vi "Initialize.vi"(8 "error in (no error)":errorcluster, 9 "Data Cluster (for Table Headers)":variant, 10 "TableLogger Config":T1, 11 "object in":refnum<class "TableLogger_SQLite_Actor.lvclass">) -> (0 "error out":errorcluster, 3 "object out":refnum<class "TableLogger_SQLite_Actor.lvclass">)   [LabVIEW 2014, in "TableLogger_SQLite_Actor.lvlib" / "TableLogger_SQLite_Actor.lvclass"]
uses:
  TableLogger_SQLite_Actor.lvclass
  TableLogger_Actor/TableLoggerConfig.ctl
  TableLogger_Actor/TableLoggerTypes.ctl
  TableLogger_Actor/TableLoggerBackupConfig.ctl
  TableLogger_SQLite_Actor.lvclass/TableLogger_SQLite_Actor.ctl
  <vilib>/drjdpowell/SQLite Library/SQL Connection/Open (path).vi
  <vilib>/drjdpowell/SQLite Library/SQL Connection/Open (string).vi
  <userlib>/_OpenG.lib/file/file.llb/Strip Path - Traditional__ogtk.vi
  <vilib>/AdvancedString/Path To Command Line String.vi
  <vilib>/drjdpowell/SQLite Library/SQL Connection/Execute SQL (No results).vi
  TableLogger_Actor/TableLogger_Actor/TableLogger_Actor.lvclass
  <vilib>/drjdpowell/SQLite Library/SQL Connection/Connection.lvclass
  <vilib>/drjdpowell/SQLite Library/SQLite.lvlib
  TableLogger_Actor/TableLogger_Actor.lvlib
panel:
  # "Connector Pane"
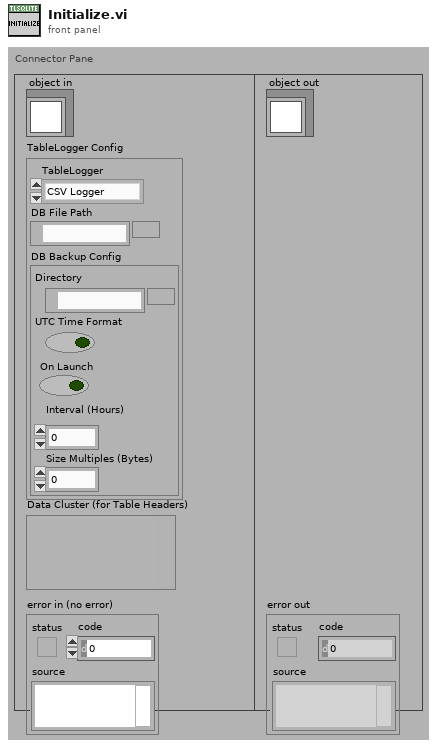
[diagram p1: front panel]
types:
  T1 = typedef "TableLogger_Actor.lvlib/TableLoggerConfig.ctl" = cluster{"TableLogger":T2, "DB File Path":path, "DB Backup Config":T3}
  T2 = typedef "TableLogger_Actor.lvlib/TableLoggerTypes.ctl" = enum16{"CSV Logger", "SQLite Logger"}
  T3 = typedef "TableLogger_Actor.lvlib/TableLoggerBackupConfig.ctl" = cluster{"Directory":path, "UTC Time Format":bool, "On Launch":bool, "Interval (Hours)":dbl, "Size Multiples (Bytes)":i32}
  T4 = typedef "Type Descriptor Enumeration__ogtk.ctl" = enum8{"<Null>", "I8", "I16", "I32", "I64", "U8", "U16", "U32", "U64", "SGL", "DBL", "EXT", "CSG", "CDB", "CXT", "0x0F", "0x10", "0x11", "0x12", "0x13", "0x14", "Enum U8", "Enum U16", "Enum U32", "Enum U64", "SGL PQ", "DBL PQ", "EXT PQ", "CSG PQ", "CDB PQ", "CXT PQ", "0x1F", "0x20", "Boolean", "0x22", "0x23", "0x24", "0x25", "0x26", "0x27", "0x28", "0x29", "0x2A", "0x2B", "0x2C", "0x2D", "0x2E", "0x2F", "String", "0x31", "Path", "Pict", "0x34", "0x35", "0x36", "DAQ", "0x38", "0x39", "0x3A", "0x3B", "0x3C", "0x3D", "0x3E", "0x3F", "Array", "0x41", "0x42", "0x43", "0x44", "0x45", "0x46", "0x47", "0x48", "0x49", "0x4A", "0x4B", "0x4C", "0x4D", "0x4E", "0x4F", "Cluster", "0x51", "0x52", "Variant", "Waveform", "0x55", "0x56", "0x57", "0x58", "0x59", "0x5A", "0x5B", "0x5C", "0x5D", "0x5E", "0x5F", "0x60", "0x61", "0x62", "0x63", "0x64", "0x65", "0x66", "0x67", "0x68", "0x69", "0x6A", "0x6B", "0x6C", "0x6D", "0x6E", "0x6F", "Refnum"}
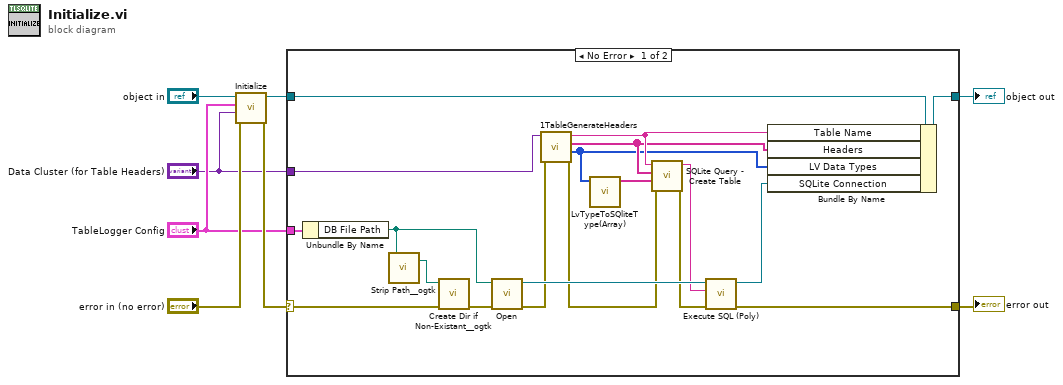
[diagram p0: block diagram]
diagram:
  n1 = call-parent "Initialize.vi"("error in (no error)"="error in (no error)", "Data Cluster (for Headers)"="Data Cluster (for Table Headers)", "TableLogger Config"="TableLogger Config", "object in"="object in") -> ("error out"=w3:errorcluster, "object out"=w5:refnum<class "TableLogger_SQLite_Actor.lvclass">)  [unwired: 6 in]
  n2 = case shown="No Error" w3 {
    selector: w3 -> [w27 w29]
    tunnel: [w22 w29] -> w8
    tunnel: [w26 w28] -> w7
    tunnel: w5 -> [w25 w28]
    tunnel: "TableLogger Config" -> [w12 _]
    tunnel: "Data Cluster (for Table Headers)" -> [w21 _]
    frame No Error {
      n3 = Unbundle By Name(w12) -> ("DB File Path"=w11:path)
      n4 = call-poly <userlib>:"Strip Path__ogtk.vi"("path"=w11) -> ("stripped path"=w9:path)  [unwired: 1 out]
      n5 = call <userlib>:"Create Dir if Non-Existant__ogtk.vi"("error in (no error)"=w27, "Directory Path"=w9) -> ("error out"=w10:errorcluster)  [unwired: 7 in, 2 out]
      n6 = call-poly <vilib>:"Open.vi"("error in (no error)"=w10, "db file"=w11) -> ("error out"=w20:errorcluster, "SQLite Connection"=w24:refnum<class "Connection.lvclass">)  [unwired: 8 in]
      n7 = call "1TableGenerateHeaders.vi"("error in (no error)"=w20, "Cluster Variant"=w21) -> ("error out"=w19:errorcluster, "LV Data Types"=w14:T4[], "Headers"=w15:string[], "Table Name"=w16:string)  [unwired: 6 in]
      n8 = call "LvTypeToSQliteType(Array).vi"("Type Descriptor Enumeration"=w14) -> ("String"=w13:string[])  [unwired: 10 in]
      n9 = call "SQLite Query - Create Table.vi"("error in"=w19, "Table Col SQL Data Types"=w13, "Table Headers"=w15, "Table Name"=w16) -> ("error out"=w17:errorcluster, "SQLite Query"=w18:string)  [unwired: 6 in]
      n10 = call-poly <vilib>:"Execute SQL (Poly).vi"("error in (no error)"=w17, "SQL"=w18, "SQLite Connection in"=w24) -> ("error out"=w22:errorcluster, "SQLite Connection"=w23:refnum<class "Connection.lvclass">)  [unwired: 7 in]
      n11 = Bundle By Name(cluster=w25, "Table Name"=w16, "Headers"=w15, "LV Data Types"=w14, "SQLite Connection"=w23) -> (w26:refnum<class "TableLogger_SQLite_Actor.lvclass">)
    }
    frame Error {
    }
  }
  "error out" <- w8
  "object out" <- w7
